vi "Add Service.vi"(8 "error in (no error)":errorcluster, 10 "Service":refnum<class "Service.lvclass">, 11 "Arguments in":refnum<class "Arguments.lvclass">) -> (0 "error out":errorcluster, 3 "Arguments out":refnum<class "Arguments.lvclass">)   [LabVIEW 2020, in "HTTP Server.lvlib" / "Arguments.lvclass"]
uses:
  Arguments.lvclass
  Arguments.lvclass/Arguments.ctl
  <vilib>/Utility/miscctls.llb/LVMapReplaceAction.ctl
  <vilib>/ErrorRing/Error Ring.xnode
  <vilib>/Utility/error.llb/Error Cluster From Error Code.vi
  Service/Service.lvclass
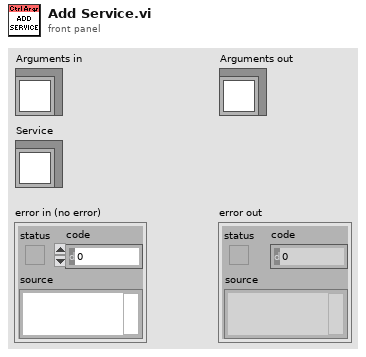
[diagram p1: front panel]
types:
  T1 = typedef "LVMapReplaceAction.ctl" = enum32{"Modify Entry only if found", "Add or Modify Entry", "Delete Entry"}
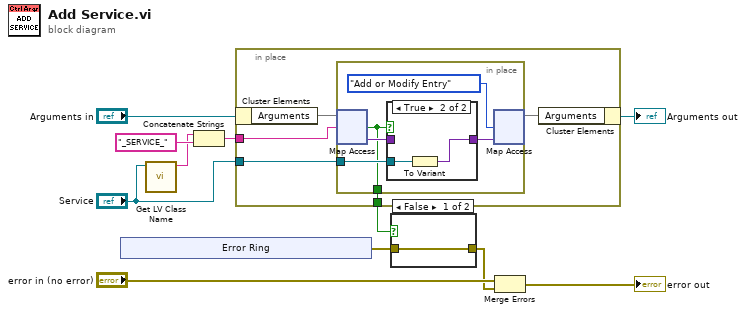
[diagram p0: block diagram]
diagram:
  n1 = xnode "Error Ring"() -> ("error out"=w4:errorcluster)
  n2 = call <vilib>:"Get LV Class Name.vi"("object"="Service") -> ("class name"=w9:string)  [unwired: 9 in, 1 out]
  n3 = Concatenate Strings(w9, "_SERVICE_" ("string")) -> (w7:string)
  n4 = in-place {
    in-place-border: w7 -> [w15]
    in-place-border: "Service" -> [w14]
    in-place-border: [w12] -> w5
    n5 = in-place-cluster #1("Arguments in") -> ("Arguments"=w16:map{string, variant})
    n6 = in-place {
      in-place-border: w14 -> [w19]
      in-place-border: [w17] -> w12
      n7 = in-place-map #2(w16, w15) -> (w20:variant, w17:bool)  [unwired: 1 in]
      n8 = case shown="True" w17 {
        tunnel: w20 -> [w22 _]
        tunnel: w19 -> [_ w24]
        tunnel: [w22 w23] -> w18
        frame False {
        }
        frame True {
          n9 = To Variant(anything=w24) -> (Variant=w23:variant)
        }
      }
      n10 = in-place-map #2(w18, LVMapReplaceAction."Add or Modify Entry" ("action")) -> (w13:map{string, variant})  [unwired: 2 out]
    }
    n11 = in-place-cluster #1("Arguments"=w13) -> (→"Arguments out":refnum<class "Arguments.lvclass">)
  }
  n12 = case shown="False" w5 {
    tunnel: w4 -> [w25 _]
    tunnel: [w25 _] -> w2
    frame False {
    }
    frame True {
    }
  }
  n13 = Merge Errors("error in (no error)", w2) -> (→"error out":errorcluster)
